vi "poor-man-crio-con-reader.vi"() -> ()   [LabVIEW 2017]
panel:
  in  "milliseconds to wait":u32=10
  in  "VISA Resource Name":refnum<visa-resource-name>="GPIB0::12::INSTR"
  out "Crio-T (K)":dbl=11.3532 format="%.5f"
  in  "stop":bool
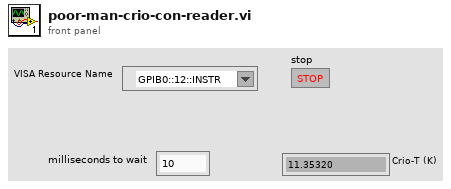
[diagram p1: front panel]
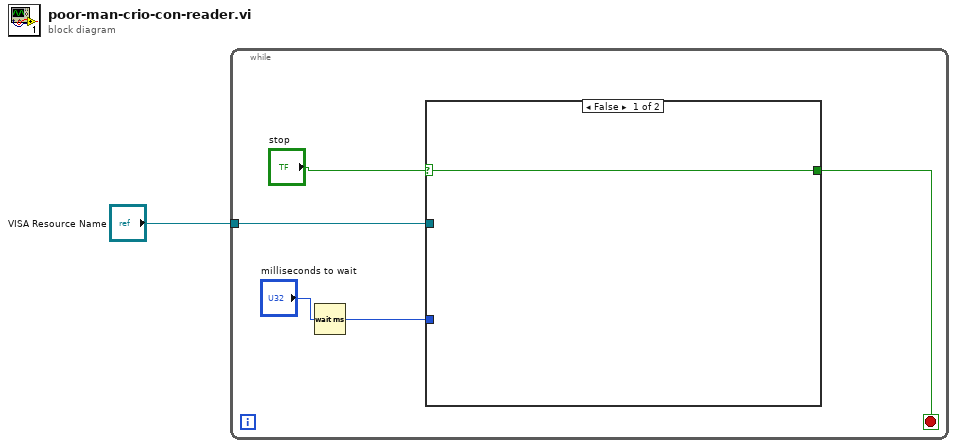
[diagram p0: block diagram]
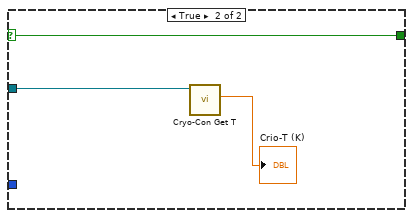
[diagram p2: hidden frame]
diagram:
  n1 = while {
    tunnel: "VISA Resource Name" -> [w6]
    stop <- w2 stop-if-true
    n2 = Wait (ms)(milliseconds to wait="milliseconds to wait") -> (millisecond timer value=w5:u32)
    n3 = case shown="False" "stop" {
      selector: "stop" -> [w7 w8]
      tunnel: w6 -> [_ w9]
      tunnel: w5 -> [_ _]
      tunnel: [w7 w8] -> w2
      frame False {
      }
      frame True {
        n4 = call "Cryo-Con Get T.vi"("VISA Resource Name"=w9) -> ("Temperature"=→"Crio-T (K)":dbl)  [unwired: 7 in, 3 out]
      }
    }
  }
